vi "Kelvinox_Split_Cluster.vi"(0 "Kelvinox-Cluster":T3 {"Sample 2" format="%_3g"; "Sorb" format="%_3g"; "MC Heater" format="%#.0f"; "Sorb Heater" format="%#.0f"; "Still Heater" format="%#.0f"; "Rate (K/min)" min=0.0 max=1.0 step=0.001 format="%.3g"; "Setpoint-Manual" min=0.0 max=10.0 step=0.001 format="%.3f"; "T-Setpoint" format="%.3f"; "Sample" format="%_3g"; "4K" format="%_3g"; "MC" format="%_3g"; "Cold\nPlate" format="%_3g"; "1K Pot" format="%_3g"; "Still" format="%_3g"; "P5" format="%_3f"; "P4" format="%_3f"; "P3" format="%_3f"; "P2" format="%_3f"; "P1" format="%_3g"; "Dump" scale=0.0..1000.0}) -> (1 "Kelvinox-Status":T1 {"Sample 2" format="%_3g"; "Sorb Heater" format="%#.0f"; "Still Heater" format="%#.0f"; "MC Heater" format="%#.0f"; "Sample" format="%_3g"; "4K" format="%_3g"; "MC" format="%_3g"; "Cold\nPlate" format="%_3g"; "1K Pot" format="%_3g"; "Still" format="%_3g"; "P5" format="%_3f"; "P4" format="%_3f"; "P3" format="%_3f"; "P2" format="%_3f"; "P1" format="%_3g"; "Dump" scale=0.0..755.0}, 2 "Kelvinox-Control":T2)   [LabVIEW 2019]
uses:
  Kelvinox/Kelvinox_Cluster.ctl
  Kelvinox/Kelvinox_Control.ctl
  Kelvinox/Kelvinox_Status.ctl
panel:
  # "Hz"
  # "Pressures in mbar"
  # "Temperatures in K"
  # "Heater Outputs in µW"
  # "DU"
  # "He\nTrap"
  # "LN2\nTrap"
  # "Pressures in mbar"
  # "Temperatures in K"
  # "Hz"
  # "Pressures in mbar"
  # "Temperatures in K"
  # "Heater Outputs\nin µW"
  # "DU"
  # "He\nTrap"
  # "LN2\nTrap"
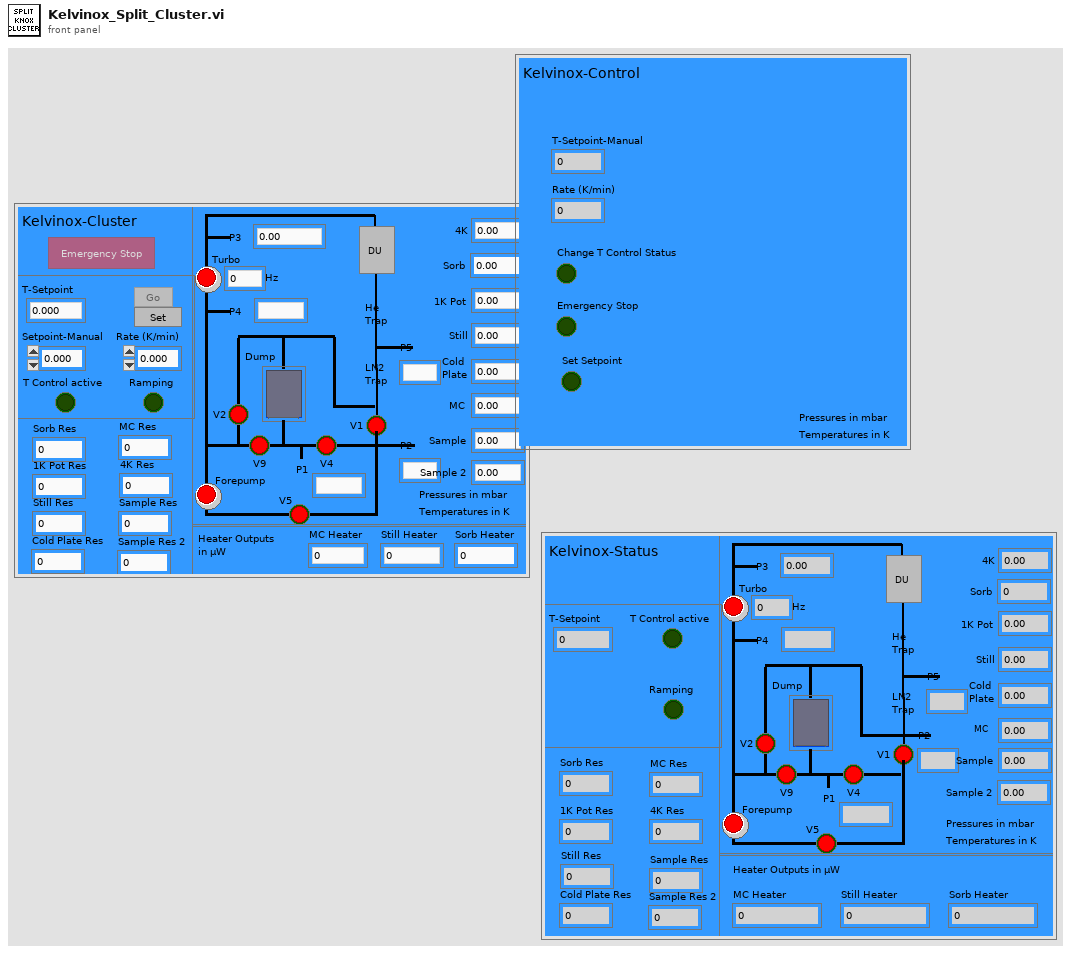
[diagram p1: front panel]
types:
  T1 = typedef "Kelvinox_Status.ctl" = cluster{"V1":bool, "V2":bool, "Dump":u16, "V4":bool, "V5":bool, "V9":bool, "P1":dbl, "P2":dbl, "P3":dbl, "P4":dbl, "P5":dbl, "Turbo":bool, "Forepump":bool, "speed":dbl, "Sorb":dbl, "1K Pot":dbl, "Still":dbl, "Cold\nPlate":dbl, "MC":dbl, "4K":dbl, "Sample":dbl, "T-Setpoint":dbl, "MC Heater":dbl, "Still Heater":dbl, "Sorb Heater":dbl, "T Control active":bool, "Sorb Res":dbl, "1K Pot Res":dbl, "Still Res":dbl, "Cold Plate Res":dbl, "MC Res":dbl, "4K Res":dbl, "Sample Res":dbl, "Ramping":bool, "Sample Res 2":dbl, "Sample 2":dbl}
  T2 = typedef "Kelvinox_Control.ctl" = cluster{"T-Setpoint-Manual":dbl, "Rate (K/min)":dbl, "Change T Control Status":bool, "Emergency Stop":bool, "Set Setpoint":bool}
  T3 = typedef "Kelvinox_Cluster.ctl" = cluster{"V1":bool, "V2":bool, "Dump":u16, "V4":bool, "V5":bool, "V9":bool, "P1":dbl, "P2":dbl, "P3":dbl, "P4":dbl, "P5":dbl, "Turbo":bool, "Forepump":bool, "speed":dbl, "Sorb":dbl, "1K Pot":dbl, "Still":dbl, "Cold\nPlate":dbl, "MC":dbl, "4K":dbl, "Sample":dbl, "T-Setpoint":dbl, "Setpoint-Manual":dbl, "Rate (K/min)":dbl, "Emergency Stop":bool, "Still Heater":dbl, "Sorb Heater":dbl, "T Control active":bool, "MC Heater":dbl, "Sorb Res":dbl, "1K Pot Res":dbl, "Still Res":dbl, "Cold Plate Res":dbl, "MC Res":dbl, "4K Res":dbl, "Sample Res":dbl, "Set Setpoint":bool, "Ramping":bool, "Change T Control Status":bool, "Sample Res 2":dbl, "Sample 2":dbl}
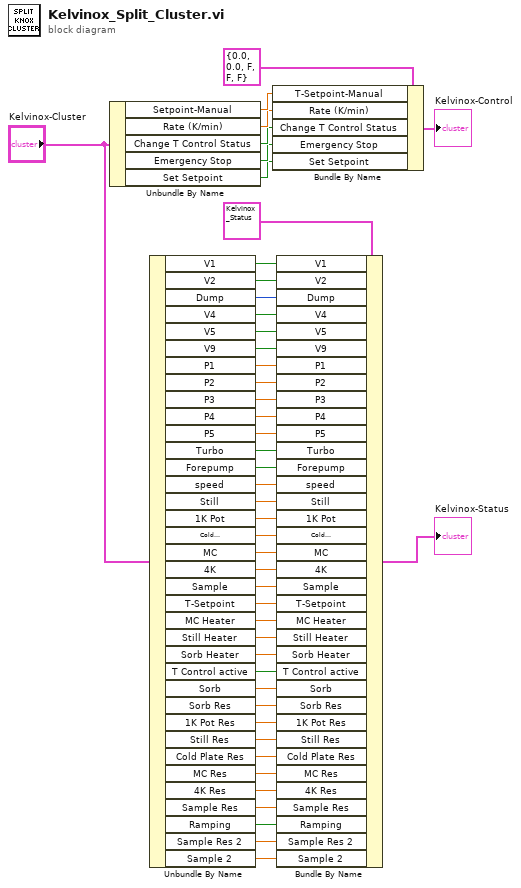
[diagram p0: block diagram]
diagram:
  n1 = Unbundle By Name("Kelvinox-Cluster") -> ("Setpoint-Manual"=w17:dbl, "Rate (K/min)"=w16:dbl, "Change T Control Status"=w15:bool, "Emergency Stop"=w14:bool, "Set Setpoint"=w4:bool)
  n2 = Unbundle By Name("Kelvinox-Cluster") -> ("V1"=w45:bool, "V2"=w44:bool, "Dump"=w43:u16, "V4"=w42:bool, "V5"=w41:bool, "V9"=w40:bool, "P1"=w39:dbl, "P2"=w38:dbl, "P3"=w37:dbl, "P4"=w36:dbl, "P5"=w35:dbl, "Turbo"=w34:bool, "Forepump"=w33:bool, "speed"=w32:dbl, "Still"=w31:dbl, "1K Pot"=w30:dbl, "Cold\nPlate"=w29:dbl, "MC"=w28:dbl, "4K"=w27:dbl, "Sample"=w26:dbl, "T-Setpoint"=w25:dbl, "MC Heater"=w24:dbl, "Still Heater"=w23:dbl, "Sorb Heater"=w22:dbl, "T Control active"=w21:bool, "Sorb"=w12:dbl, "Sorb Res"=w11:dbl, "1K Pot Res"=w10:dbl, "Still Res"=w9:dbl, "Cold Plate Res"=w8:dbl, "MC Res"=w7:dbl, "4K Res"=w6:dbl, "Sample Res"=w5:dbl, "Ramping"=w3:bool, "Sample Res 2"=w2:dbl, "Sample 2"=w1:dbl)
  n3 = Bundle By Name(cluster=T2 {"T-Setpoint-Manual"=0.0, "Rate (K/min)"=0.0, "Change T Control Status"=FALSE, "Emergency Stop"=FALSE, "Set Setpoint"=FALSE} ("Kelvinox-Cluster"), "T-Setpoint-Manual"=w17, "Rate (K/min)"=w16, "Change T Control Status"=w15, "Emergency Stop"=w14, "Set Setpoint"=w4) -> (→"Kelvinox-Control":T2)
  n4 = Bundle By Name(cluster=T1 {"V1"=FALSE, "V2"=FALSE, "Dump"=0, "V4"=FALSE, "V5"=FALSE, "V9"=FALSE, "P1"=0.0, "P2"=0.0, "P3"=0.0, "P4"=0.0, "P5"=0.0, "Turbo"=FALSE, "Forepump"=FALSE, "speed"=0.0, "Sorb"=0.0, "1K Pot"=0.0, "Still"=0.0, "Cold\nPlate"=0.0, "MC"=0.0, "4K"=0.0, "Sample"=0.0, "T-Setpoint"=0.0, "MC Heater"=0.0, "Still Heater"=0.0, "Sorb Heater"=0.0, "T Control active"=FALSE, "Sorb Res"=0.0, "1K Pot Res"=0.0, "Still Res"=0.0, "Cold Plate Res"=0.0, "MC Res"=0.0, "4K Res"=0.0, "Sample Res"=0.0, "Ramping"=FALSE, "Sample Res 2"=0.0, "Sample 2"=0.0} ("Kelvinox-Cluster"), "V1"=w45, "V2"=w44, "Dump"=w43, "V4"=w42, "V5"=w41, "V9"=w40, "P1"=w39, "P2"=w38, "P3"=w37, "P4"=w36, "P5"=w35, "Turbo"=w34, "Forepump"=w33, "speed"=w32, "Still"=w31, "1K Pot"=w30, "Cold\nPlate"=w29, "MC"=w28, "4K"=w27, "Sample"=w26, "T-Setpoint"=w25, "MC Heater"=w24, "Still Heater"=w23, "Sorb Heater"=w22, "T Control active"=w21, "Sorb"=w12, "Sorb Res"=w11, "1K Pot Res"=w10, "Still Res"=w9, "Cold Plate Res"=w8, "MC Res"=w7, "4K Res"=w6, "Sample Res"=w5, "Ramping"=w3, "Sample Res 2"=w2, "Sample 2"=w1) -> (→"Kelvinox-Status":T1)
